vi "Main.vi"(8 "error in (no error)":errorcluster) -> (0 "error out":errorcluster)   [LabVIEW 2014, in "Error Module.lvlib"]
uses:
  Error Module.lvlib
  Queue FGV.ctl
  Message.ctl
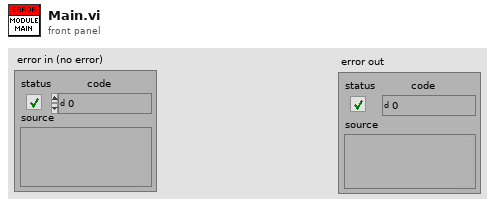
[diagram p1: front panel]
types:
  T1 = typedef "Error Module.lvlib/Queue FGV.ctl" = enum16{"Set", "Get", "Release"}
  T2 = typedef "Error Module.lvlib/Message.ctl" = cluster{"Message":enum16{"Initialise", "Error", "Close"}, "Data":variant}
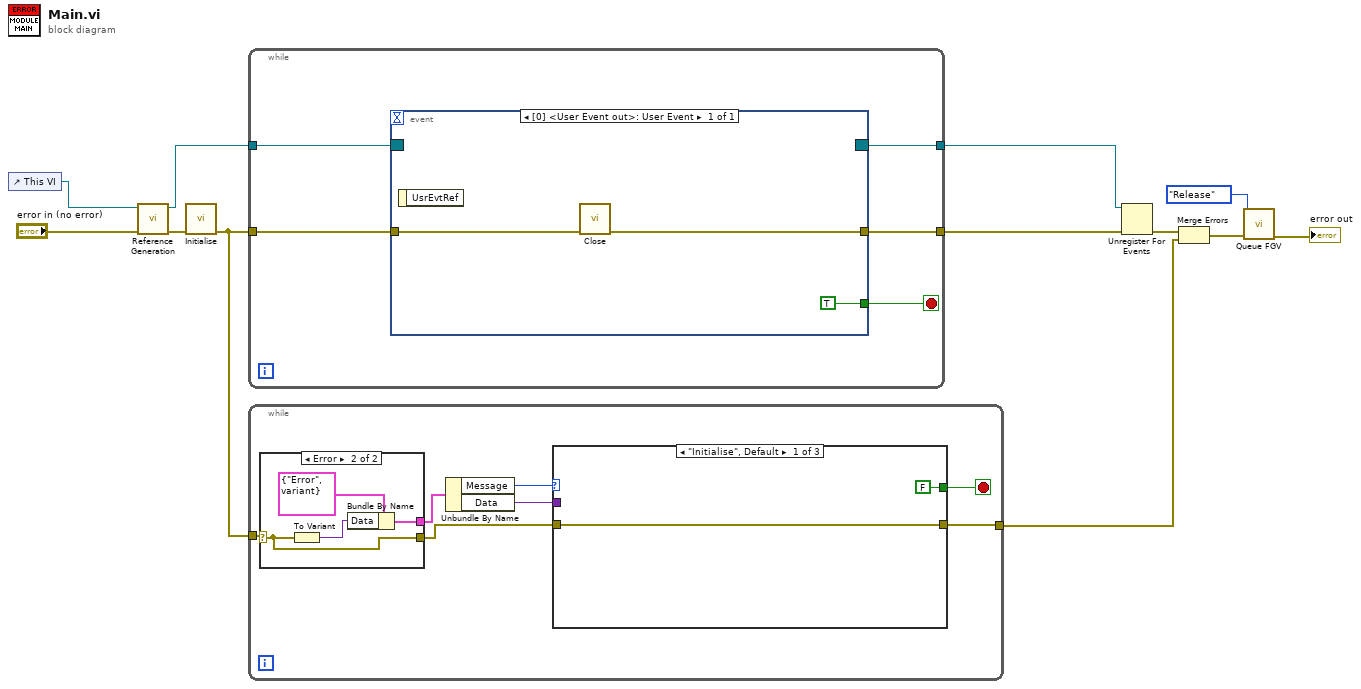
[diagram p0: block diagram]
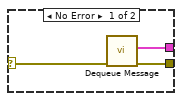
[diagram p2: hidden frame]
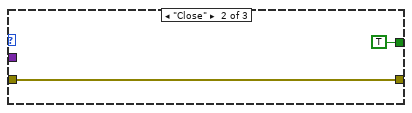
[diagram p3: hidden frame]
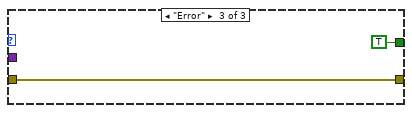
[diagram p4: hidden frame]
diagram:
  n1 = control-ref of="This VI"() -> (w12:refnum<vi>)
  n2 = call "Reference Generation.vi"("error in (no error)"="error in (no error)", "VI in"=w12) -> ("error out"=w10:errorcluster, "User Events Reference"=w9:refnum<event-registration>)  [unwired: 8 in]
  n3 = call "Initialise.vi"("error in (no error)"=w10) -> ("error out"=w8:errorcluster)  [unwired: 10 in]
  n4 = while {
    tunnel: w9 -> [w17]
    tunnel: w8 -> [w16]
    tunnel: [w14] -> w7
    tunnel: [w13] -> w6
    stop <- w15 stop-if-true
    n5 = event shown="[0] <User Event out>: User Event" {
      selector: w17 -> [_]
      dyn-events: [_] -> w14
      timeout: _ -> [_]
      tunnel: w16 -> [w20]
      tunnel: [TRUE] -> w15
      tunnel: [w18] -> w13
      event User Event {
        n6 = event-data() -> ()  [unwired: 1 in, 1 out]
        n7 = call "Close.vi"("error in (no error)"=w20) -> ("error out"=w18:errorcluster)  [unwired: 10 in]
      }
    }
  }
  n8 = while {
    tunnel: w8 -> [w26]
    tunnel: [w21] -> w5
    stop <- w23 stop-if-true
    n9 = case shown="Error" w26 {
      selector: w26 -> [w30 w33]
      tunnel: [w29 w33] -> w24
      tunnel: [w28 w31] -> w22
      frame No Error {
        n10 = call "Dequeue Message.vi"("error in (no error)"=w30) -> ("error out"=w29:errorcluster, "output cluster"=w28:T2)  [unwired: 8 in, 1 out]
      }
      frame Error {
        n11 = To Variant(anything=w33) -> (Variant=w32:variant)
        n12 = Bundle By Name(cluster=T2 {"Message"=enum."Error", "Data"=variant} ("output cluster"), "Data"=w32) -> (w31:T2)
      }
    }
    n13 = Unbundle By Name(w22) -> ("Message"=w27:enum16{"Initialise", "Error", "Close"}, "Data"=w25:variant)
    n14 = case shown="\"Initialise\", Default" w27 {
      tunnel: w25 -> [_ _ _]
      tunnel: w24 -> [w36 w38 w39]
      tunnel: [w36 w38 w39] -> w21
      tunnel: [FALSE ("event data") TRUE ("event data") TRUE ("event data")] -> w23
      frame "Initialise", Default {
      }
      frame "Close" {
      }
      frame "Error" {
      }
    }
  }
  n15 = Unregister For Events(event registration refnum=w7, error in=w6) -> (error out=w4:errorcluster)
  n16 = Merge Errors(w4, w5) -> (w3:errorcluster)
  n17 = call "Queue FGV.vi"("error in (no error)"=w3, "Action"=Queue_FGV."Release") -> ("error out"=→"error out":errorcluster)  [unwired: 8 in, 1 out]
